vi "Robot globals (robot acquires video).vi"() -> ()   [LabVIEW 2012]
doc: "Global variables used to define robot properties and the stop state."
panel:
  in  "Connection timeout":i32=5000
  in  "Safety commands reader name":string="Safety commands reader"
  in  "Video writer endpoint name":string="Video writer"
  in  "Robot UDP listen port":u16=60200
  in  "Video timeout":i32=5000
  in  "Robot initialization timeout":i32=-1
  in  "Runtime timeout":i32=1000
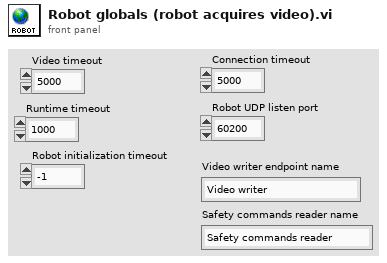
[diagram p1: front panel]
diagram:
